vi "Rebuild Frame Settings.vi"(8 "error in (no error)":errorcluster, 10 "Frames":T4(array[cluster]) {"Frame Transmit Info"."Transmit Time" format="%#_p"}, 11 "Ref in":T1 format="%.0x") -> (0 "error out":errorcluster, 3 "Ref out":T1 format="%.0x")   [LabVIEW 2013, in "J1939 Addon System Explorer.lvlib"]
uses:
  J1939 Addon System Explorer.lvlib
  Shared/Types/XNET Frame Event Properties.ctl
  Shared/Types/SPN Properties.ctl
  <vilib>/NI Veristand/Custom Device API/Custom Device Item Ref.ctl
  <vilib>/NI Veristand/Custom Device API/Custom Device Channel.ctl
  <vilib>/NI Veristand/Custom Device API/Custom Device Channel Type.ctl
  Shared/SubVIs/Constants.vi
  <vilib>/NI Veristand/Custom Device API/Set Item Property (Variant).vi
  Shared/J1939 Addon Shared.lvlib
  <vilib>/NI Veristand/Custom Device API/Custom Device API.lvlib
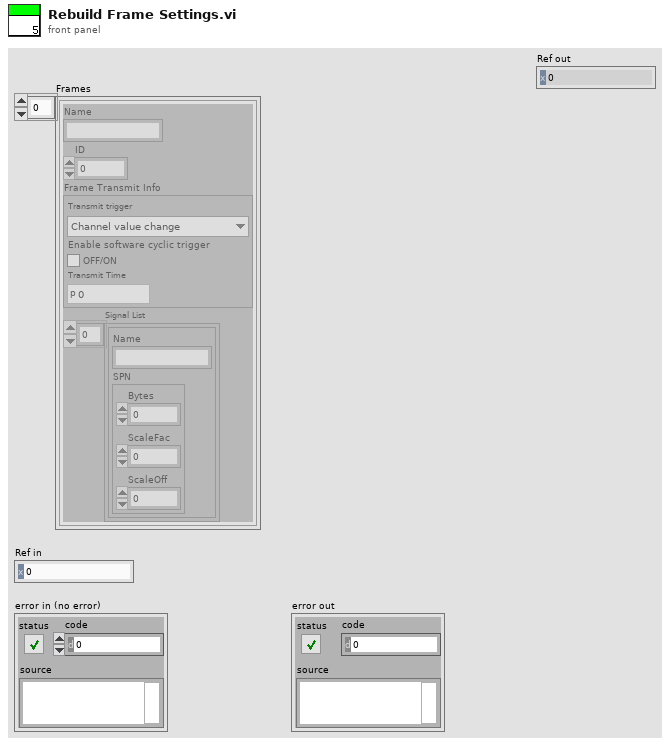
[diagram p1: front panel]
types:
  T1 = typedef "Custom Device API.lvlib/Custom Device Item Ref.ctl" = u64
  T2 = typedef "J1939 Addon Shared.lvlib/XNET Frame Event Properties.ctl" = cluster{"Transmit trigger":enum16{"Channel value change"}, "Enable software cyclic trigger":bool, "Transmit Time":dbl}
  T3 = typedef "J1939 Addon Shared.lvlib/SPN Properties.ctl" = cluster{"Bytes":u32, "ScaleFac":dbl, "ScaleOff":dbl}
  T4 = cluster{"Name":string, "ID":u32, "Frame Transmit Info":T2, "Signal List":cluster{"Name":string, "SPN":T3}[]}[]
  T5 = typedef "Custom Device API.lvlib/Custom Device Channel.ctl" = cluster{"Type":T6, "Units":string, "Default Value":dbl, "Faultable":bool, "Scalable":bool}
  T6 = typedef "Custom Device API.lvlib/Custom Device Channel Type.ctl" = enum16{"Input", "Output"}
  T7 = typedef "Custom Device API.lvlib/Custom Device Item Info.ctl" = cluster{"Name":string, "Is Channel":bool, "GUID":string, "Is Waveform":bool}
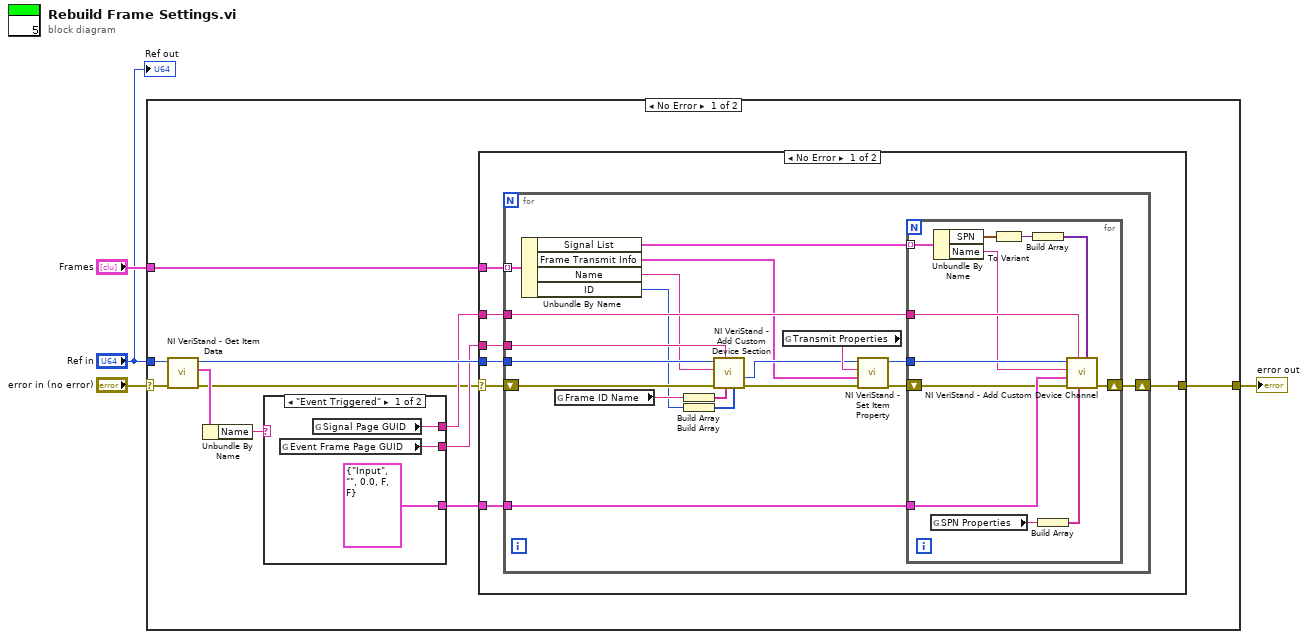
[diagram p0: block diagram]
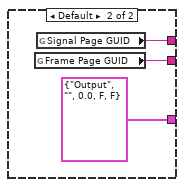
[diagram p2: hidden frame]
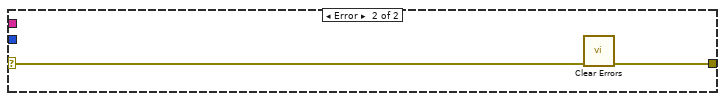
[diagram p3: hidden frame]
diagram:
  n1 = case shown="No Error" "error in (no error)" {
    selector: "error in (no error)" -> [w14 w62]
    tunnel: [w15 w62] -> w1
    tunnel: "Ref in" -> [w13 _]
    tunnel: "Frames" -> [w12 _]
    frame No Error {
      n2 = call <vilib>:"NI VeriStand - Get Item Data.vi"("error in (no error)"=w14, "Item Ref in"=w13) -> ("error out"=w5:errorcluster, "Item Info"=w10:T7, "Item Ref out"=w11:T1)  [unwired: 7 out]
      n3 = Unbundle By Name(w10) -> ("Name"=w9:string)
      n4 = case shown="\"Event Triggered\"" w9 {
        tunnel: [w18 w21] -> w8
        tunnel: [w17 w20] -> w7
        tunnel: [T5 {"Type"=enum."Input", "Units"="", "Default Value"=0.0, "Faultable"=FALSE, "Scalable"=FALSE} ("Channel") T5 {"Type"=enum."Output", "Units"="", "Default Value"=0.0, "Faultable"=FALSE, "Scalable"=FALSE} ("Channel")] -> w6
        frame "Event Triggered" {
          n5 = global read "Constants.vi" "Event Frame Page GUID"() -> (w17:string)
          n6 = global read "Constants.vi" "Signal Page GUID"() -> (w18:string)
        }
        frame Default {
          n7 = global read "Constants.vi" "Frame Page GUID"() -> (w20:string)
          n8 = global read "Constants.vi" "Signal Page GUID"() -> (w21:string)
        }
      }
      n9 = case shown="No Error" w5 {
        selector: w5 -> [w26 w61]
        tunnel: [w28 w60] -> w15
        tunnel: w11 -> [w27 _]
        tunnel: w8 -> [w25 _]
        tunnel: w7 -> [w24 _]
        tunnel: w6 -> [w23 _]
        tunnel: w12 -> [w22 _]
        frame No Error {
          n10 = for {
            shift-right: [w47] -> w28
            shift-left: w26 -> [w32]
            tunnel: w27 -> [w46]
            tunnel: w25 -> [w44]
            tunnel: w24 -> [w43]
            tunnel: w23 -> [w41]
            tunnel: w22 -> [w33] mode=indexing
            n11 = Unbundle By Name(w33) -> ("Signal List"=w34:cluster{"Name":string, "SPN":T3}[], "Frame Transmit Info"=w31:T2, "Name"=w29:string, "ID"=w30:u32)
            n12 = global read "Constants.vi" "Frame ID Name"() -> (w45:string)
            n13 = Build Array(w45) -> (w37:string[])
            n14 = Build Array(w30) -> (w38:u32[])
            n15 = call <vilib>:"NI VeriStand - Add Custom Device Section.vi"("Property Values"=w38, "Property names"=w37, "GUID (Default Section)"=w43, "error in (no error)"=w32, "Section Name"=w29, "Parent Ref in"=w46) -> ("error out"=w36:errorcluster, "Section Ptr"=w35:T1)  [unwired: 2 in, 2 out]
            n16 = global read "Constants.vi" "Transmit Properties"() -> (w42:string)
            n17 = call-poly <vilib>:"NI VeriStand - Set Item Property.vi"("error in (no error)"=w36, "Value"=w31, "Property Name"=w42, "Item Ref in"=w35) -> ("error out"=w40:errorcluster, "Item Ref out"=w39:T1)  [unwired: 5 in, 1 out]
            n18 = for {
              tunnel: w44 -> [w58]
              tunnel: w41 -> [w57]
              tunnel: w39 -> [w55]
              shift-right: [w59] -> w47
              shift-left: w40 -> [w56]
              tunnel: w34 -> [w54] mode=indexing
              n19 = global read "Constants.vi" "SPN Properties"() -> (w49:string)
              n20 = Unbundle By Name(w54) -> ("SPN"=w53:T3, "Name"=w50:string)
              n21 = To Variant(anything=w53) -> (Variant=w52:variant)
              n22 = Build Array(w52) -> (w51:variant[])
              n23 = Build Array(w49) -> (w48:string[])
              n24 = call <vilib>:"NI VeriStand - Add Custom Device Channel.vi"("Property Values"=w51, "Property names"=w48, "GUID (Default Channel)"=w58, "error in (no error)"=w56, "Channel"=w57, "Channel Name"=w50, "Parent Ref in"=w55) -> ("error out"=w59:errorcluster)  [unwired: 1 in, 3 out]
            }
          }
        }
        frame Error {
          n25 = call <vilib>:"Clear Errors.vi"("error in (no error)"=w61) -> ("error out"=w60:errorcluster)  [unwired: 6 in]
        }
      }
    }
    frame Error {
    }
  }
  "error out" <- w1
  "Ref out" <- "Ref in"
